vi "TPNT_FormatLog.vi"(9 "time in":u32, 10 "testpoint In":T1={"name"="", "type"="", "algor"=[], "update_rate"=0.0, "Limits"={"Alarm Type"="", "Lower "=0.0, "Upper"=0.0, "Nominal"=0.0, "outrange"=FALSE, "Check"=TRUE, "latch"=FALSE, "level"=""}, "Samples"={"samples"=0, "counter"=0, "Values"=[], "Current Value"="", "filter"="", "precision"=2}, "next_update"=0, "Status"="", "monitor"=TRUE, "error"=FALSE, "Log"={"log"=FALSE, "file"=path "", "type"="", "format"="", "updaterate"=0.0, "nex_update"=0, "mode"=""}, "permissions"="", "ID"=""} {"Log"."updaterate" format="%.2f"; "Samples"."Values" format="%.2f"; "Samples"."samples" min=1 step=1; "Limits"."Nominal" format="%.2f"; "Limits"."Upper" format="%.2f"; "Limits"."Lower" format="%.2f"; "update_rate" format="%.2f"}) -> (1 "message to log":string, 2 "LOG?":bool, 4 "by alarm":bool)   [LabVIEW 2016]
uses:
  TPNT_TP.ctl
  TPNT_Limits.ctl
  TPNT_Samples.ctl
  TPNT_Log.ctl
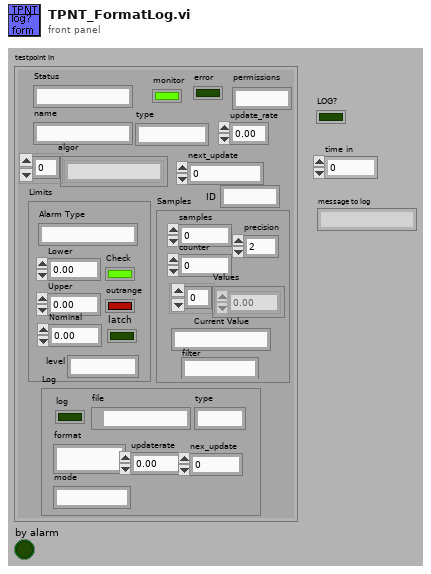
[diagram p1: front panel]
types:
  T1 = typedef "TPNT_TP.ctl" = cluster{"name":string, "type":string, "algor":string[], "update_rate":sgl, "Limits":T2, "Samples":T3, "next_update":u32, "Status":string, "monitor":bool, "error":bool, "Log":T4, "permissions":string, "ID":string}
  T2 = typedef "TPNT_Limits.ctl" = cluster{"Alarm Type":string, "Lower ":dbl, "Upper":dbl, "Nominal":dbl, "outrange":bool, "Check":bool, "latch":bool, "level":string}
  T3 = typedef "TPNT_Samples.ctl" = cluster{"samples":i32, "counter":i32, "Values":dbl[], "Current Value":string, "filter":string, "precision":u8}
  T4 = typedef "TPNT_Log.ctl" = cluster{"log":bool, "file":path, "type":string, "format":string, "updaterate":dbl, "nex_update":u32, "mode":string}
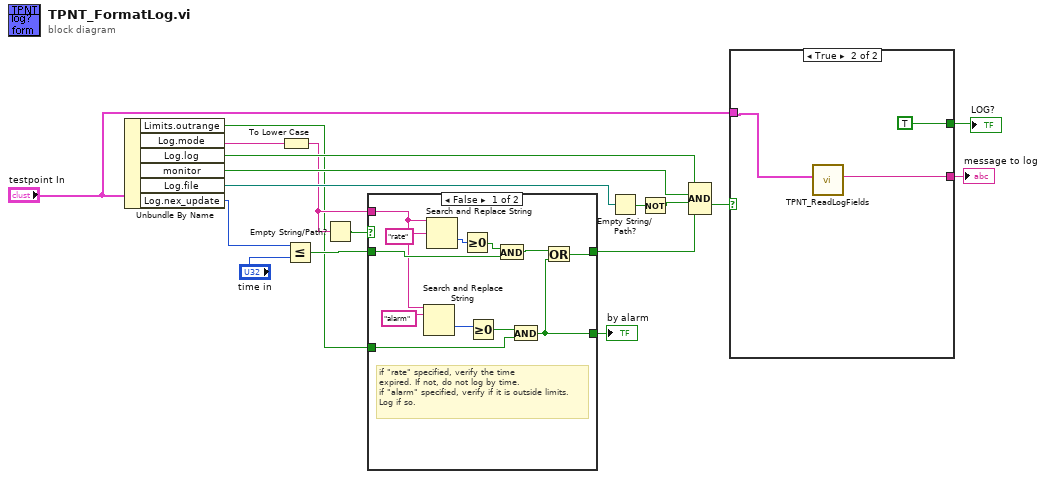
[diagram p0: block diagram]
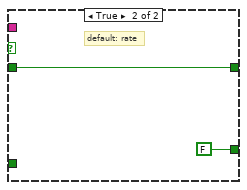
[diagram p2: hidden frame]
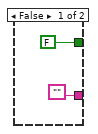
[diagram p3: hidden frame]
diagram:
  n1 = Unbundle By Name("testpoint In") -> ("Limits.outrange"=w3:bool, "Log.mode"=w8:string, "Log.log"=w18:bool, "monitor"=w17:bool, "Log.file"=w15:path, "Log.nex_update"=w13:u32)
  n2 = To Lower Case(string=w8) -> (all lower case string=w4:string)
  n3 = Less Or Equal?(x=w13, y="time in") -> (x <= y?=w6:bool)
  n4 = Empty String/Path?(string/path=w4) -> (empty?=w7:bool)
  n5 = case shown="False" w7 {
    tunnel: w6 -> [w27 w32]
    tunnel: [w20 w32] -> w5
    tunnel: w4 -> [w24 _]
    tunnel: w3 -> [w21 _]
    tunnel: [w19 FALSE] -> w1
    frame False {
      # "if \"rate\" specified, verify the time\nexpired. If not, do not log by time.\nif \"alarm\" specified, verify if it is outside limits.\nLog if so."
      n6 = Search and Replace String(input string=w24, search string="alarm") -> (offset past replacement=w26:i32)  [unwired: 1 in, 8 out]
      n7 = Search and Replace String(input string=w24, search string="rate") -> (offset past replacement=w29:i32)  [unwired: 1 in, 8 out]
      n8 = Greater Or Equal To 0?(x=w29) -> (x >= 0?=w28:bool)
      n9 = Greater Or Equal To 0?(x=w26) -> (x >= 0?=w22:bool)
      n10 = And(x=w28, y=w27) -> (x .and. y?=w23:bool)
      n11 = And(x=w22, y=w21) -> (x .and. y?=w19:bool)
      n12 = Or(x=w23, y=w19) -> (x .or. y?=w20:bool)
    }
    frame True {
      # "default: rate"
    }
  }
  "by alarm" <- w1
  n13 = Empty String/Path?(string/path=w15) -> (empty?=w16:bool)
  n14 = Not(x=w16) -> (.not. x?=w14:bool)
  n15 = Compound Arithmetic op=AND(w18, w17, w14, w5) -> (w11:bool)
  n16 = case shown="True" w11 {
    tunnel: "testpoint In" -> [_ w37]
    tunnel: ["" w36] -> w10
    tunnel: [FALSE TRUE] -> w9
    frame False {
    }
    frame True {
      n17 = call "TPNT_ReadLogFields.vi"("TPNT_TP"=w37) -> ("message to log"=w36:string)  [unwired: 1 in, 9 out]
    }
  }
  "LOG?" <- w9
  "message to log" <- w10
